vi "Time2Samples.vi"(2 "Time":dbl format="%#_6p", 3 "SampleRate":dbl format="%#_6p") -> (1 "Samples":dbl)   [LabVIEW 2013]
doc: "Converts the time duration to number of samples based on the given sample rate.\nFor writing waveforms to AWG we have to provide Even number of Samples."
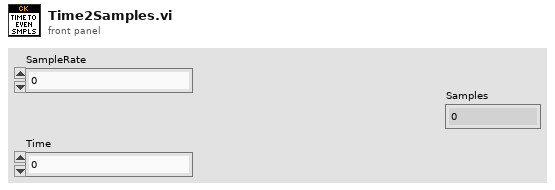
[diagram p1: front panel]
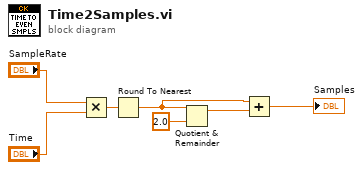
[diagram p0: block diagram]
diagram:
  n1 = Multiply(x="SampleRate", y="Time") -> (x*y=w5:dbl)
  n2 = Round To Nearest(number=w5) -> (nearest integer value=w2:dbl)
  n3 = Quotient & Remainder(x=w2, y=2.0) -> (x-y*floor(x/y)=w3:dbl)  [unwired: 1 out]
  n4 = Add(x=w2, y=w3) -> (x+y=→"Samples":dbl)
